vi "Graphe_XY.vi"(0 "Graphe":T1(graph), 3 "Tableau de chaînes":string[](array[string])) -> ()   [LabVIEW 2015]
uses:
  <vilib>/Utility/miscctls.llb/LVPositionTypeDef.ctl
panel:
  out "Calculs maths":dbl[](array[numeric])
  in  "Bouton Aide":bool
  in  "=":string
  in  "Selec Maths":u16(ring) caption="Maintenir la touche CTRL appuyée pour tout afficher" items=["Moyenne", "Min", "Max", "Ecart type", "Variance", "Intégrale", "Pente ajust. lin.", "Offset ajust. lin.", "Résidus ajust. lin.", "R²", "Amplitude ajust. exp", "Atténuation ajust. exp", "Offset ajust. exp", "Résidus ajust. exp"]
  in  "Active maths":bool
  out "Valeur maths":dbl
  out "Nbre courbes":i32
  in  "Quitter graphe":bool
  in  "Palette:Outil actif":i32
  in  "Curseur visible":bool
  in  "Tout sélectionner":bool
  in  "Curseur":u16(ring) items=["2", "3", "4", "5", "6", "7", "8"]
  in  "Quadrillage":u16(ring)=1 items=["Sans", "Horizontal", "Vertical", "Tout"]
  in  "Mini":dbl max=19.999 format="%#.3f"
  in  "Maxi":dbl min=0.001 format="%#.3f"
  in  "Echelle Y":u16(ring) items=["Manu"=0, "Auto"=2]
  out "Y":dbl
  out "X":timestamp format="%<%.3X>T"
  # "="
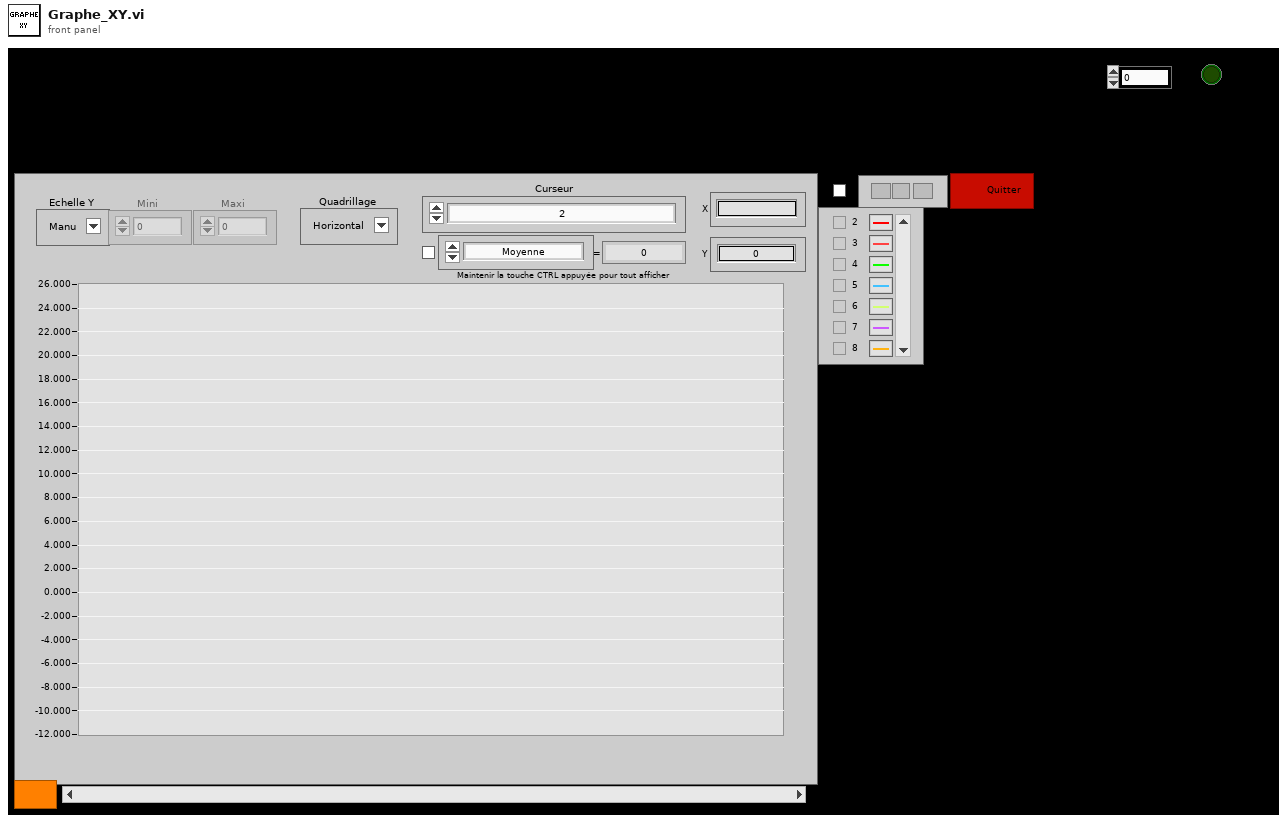
[diagram p1: front panel]
types:
  T1 = cluster{"Horodatage":timestamp[], "Donnees":dbl[]}[]
  T2 = typedef "LVPositionTypeDef.ctl" = cluster{"Left":i32, "Top":i32}
  T3 = cluster{"Shift":bool, "Ctrl":bool, "Alt":bool, "Cmd":bool, "Opt":bool}
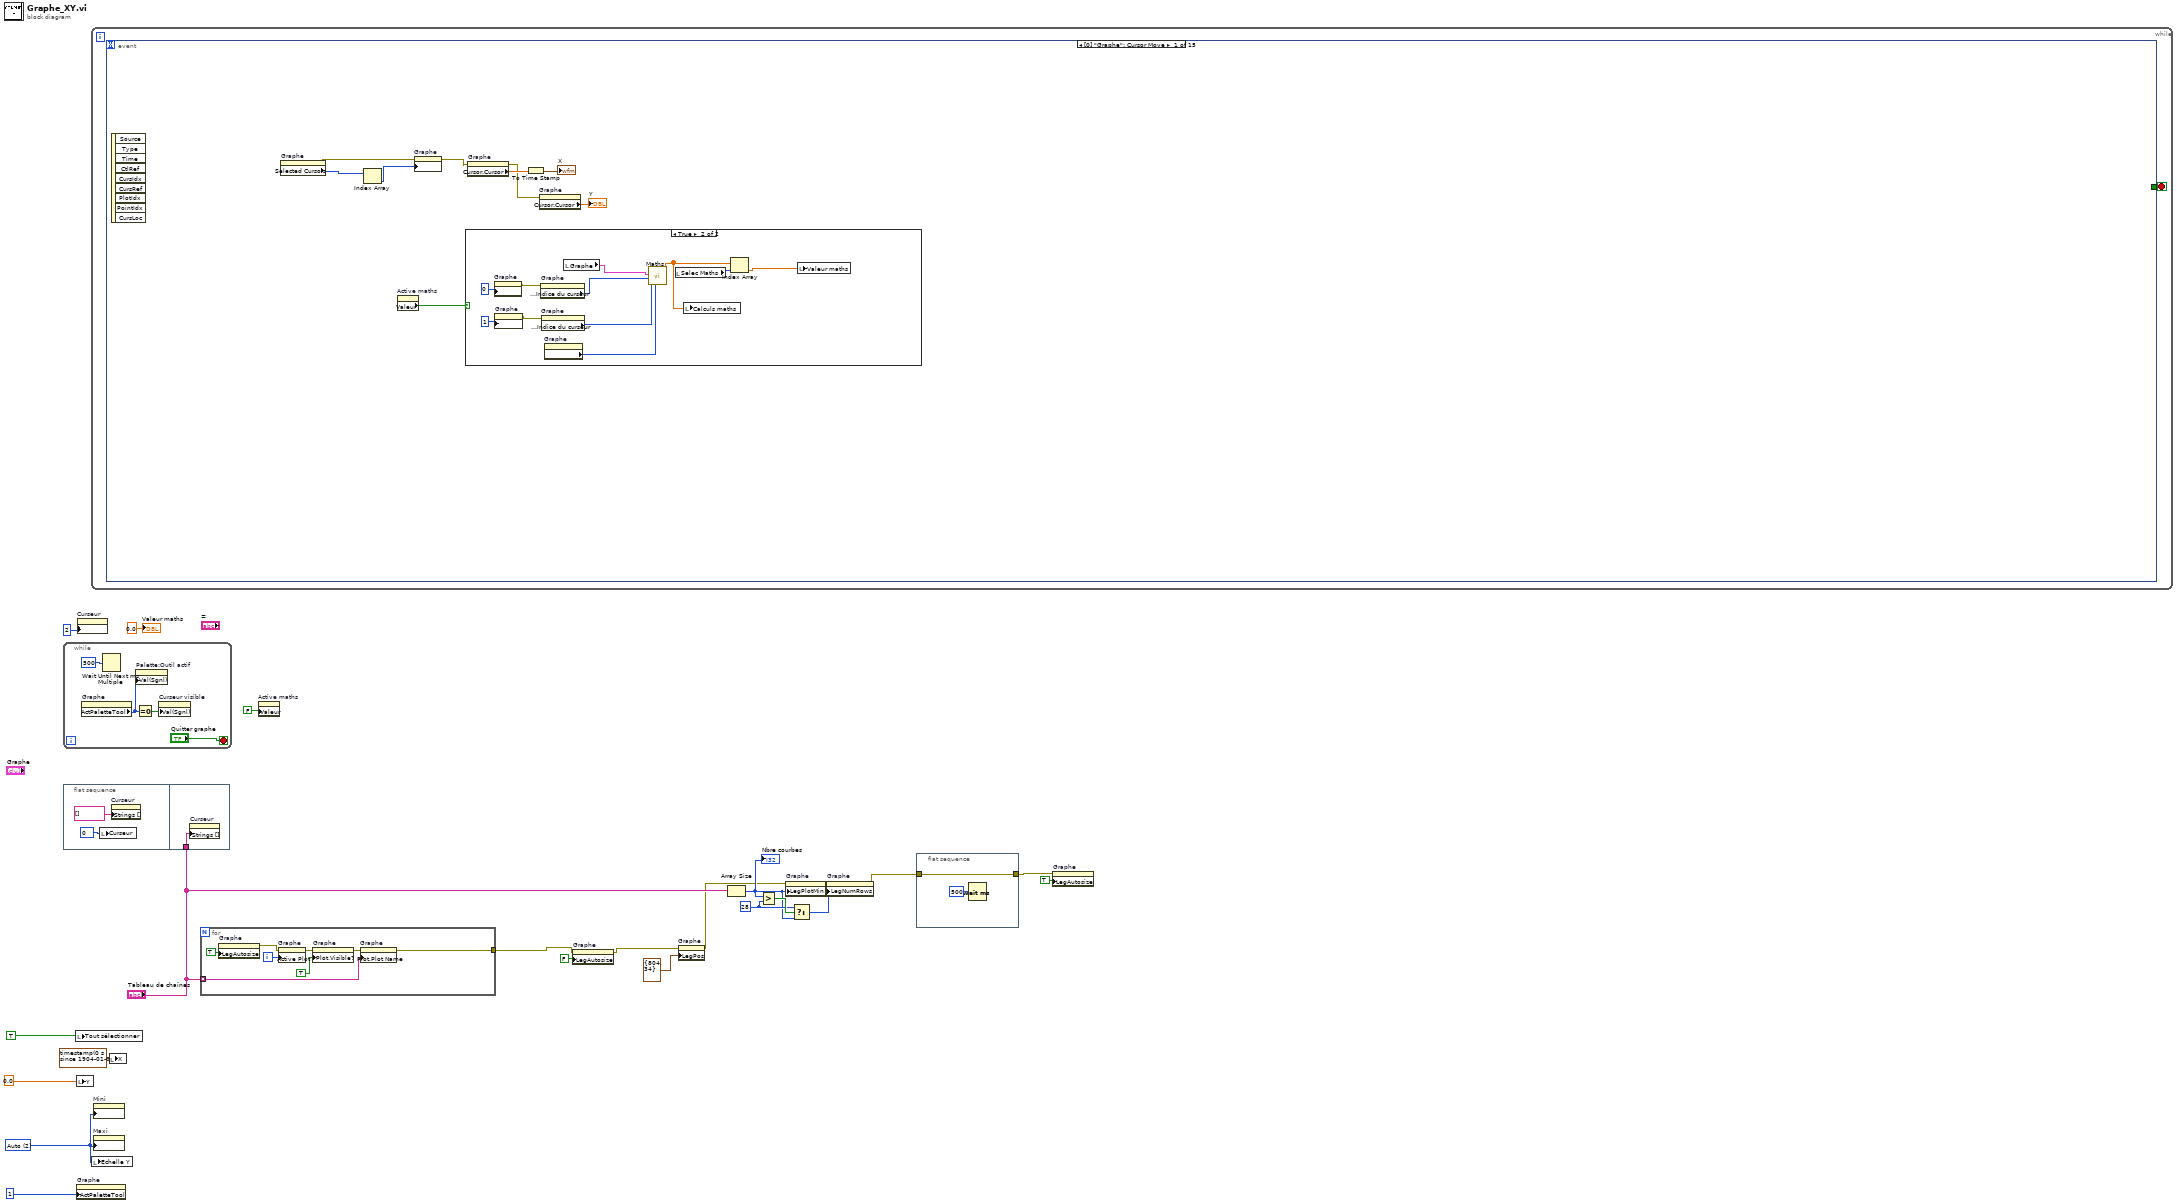
[diagram p0: block diagram]
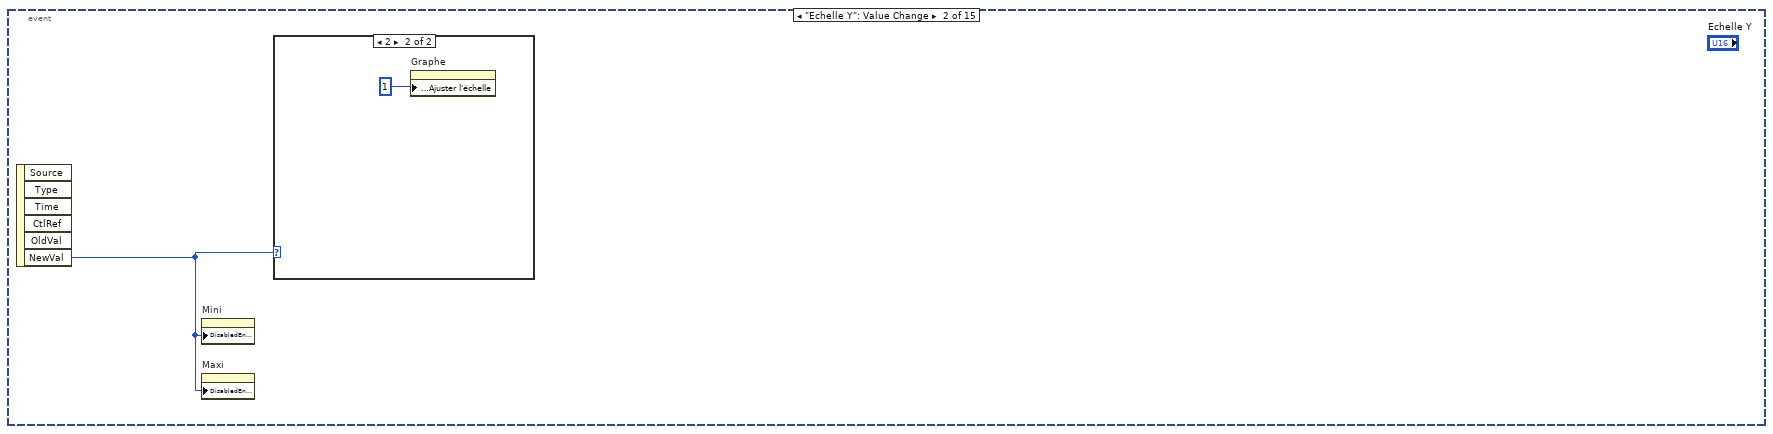
[diagram p3: hidden frame]
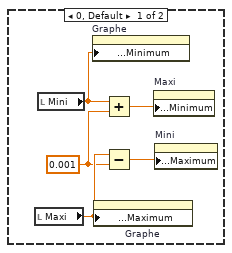
[diagram p4: hidden frame]
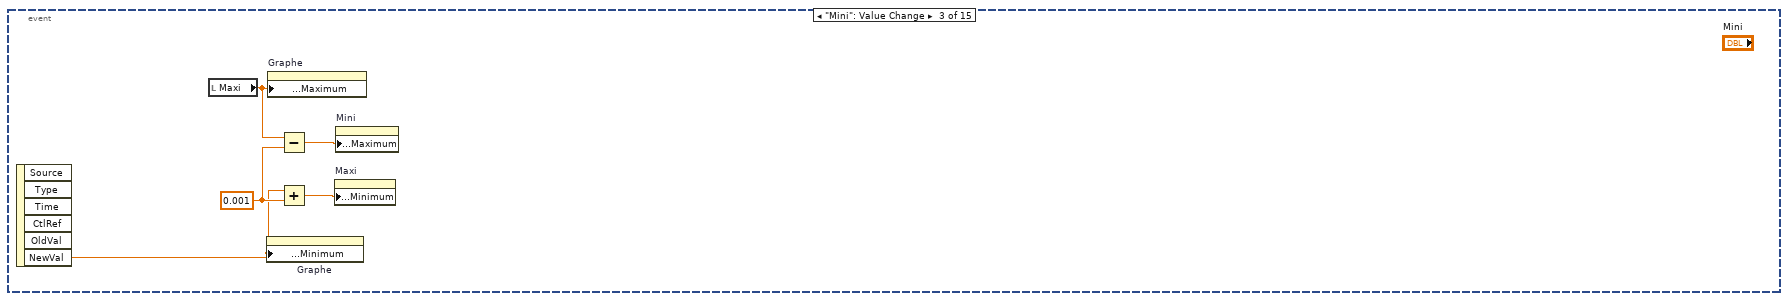
[diagram p5: hidden frame]
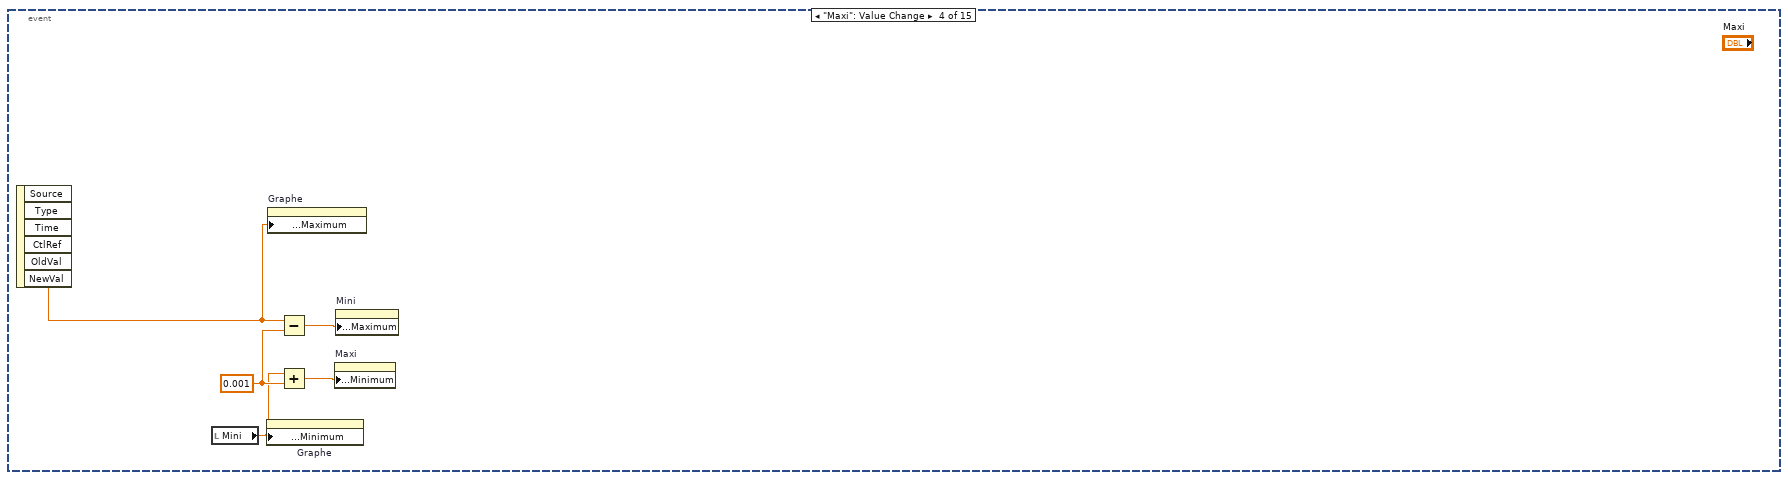
[diagram p6: hidden frame]
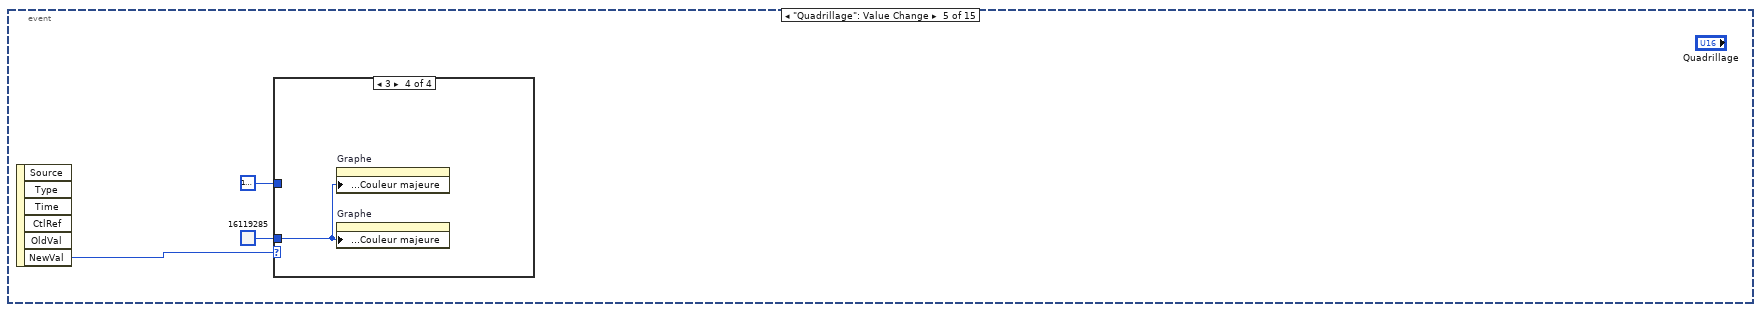
[diagram p7: hidden frame]
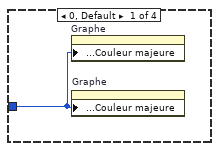
[diagram p8: hidden frame]
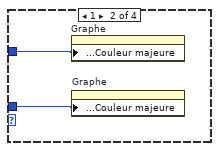
[diagram p9: hidden frame]
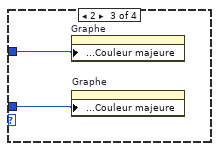
[diagram p10: hidden frame]
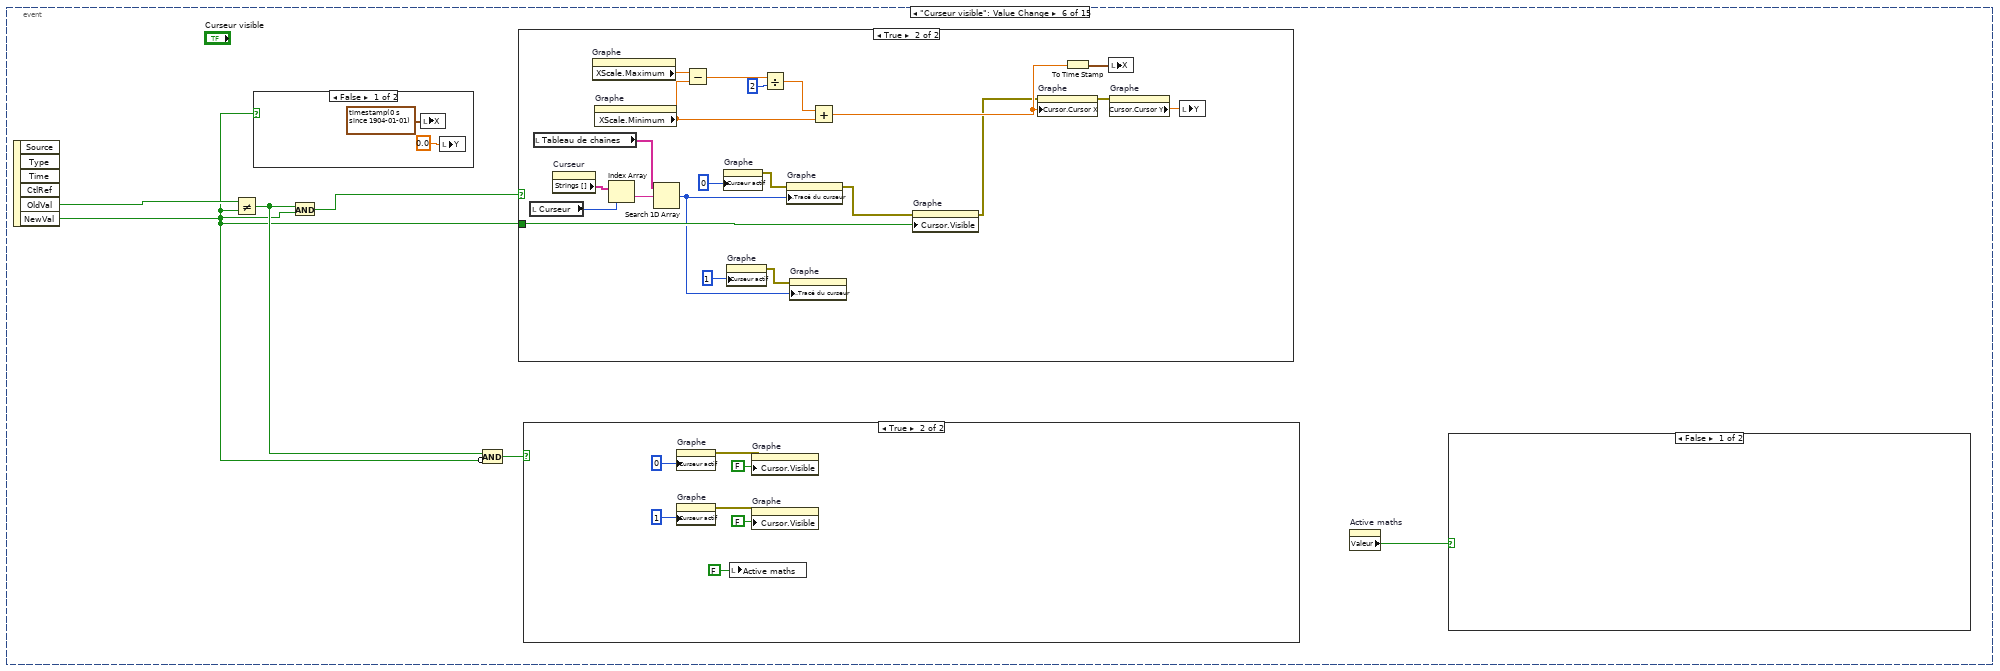
[diagram p11: hidden frame]
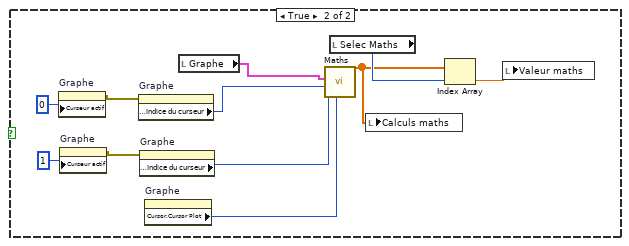
[diagram p12: hidden frame]
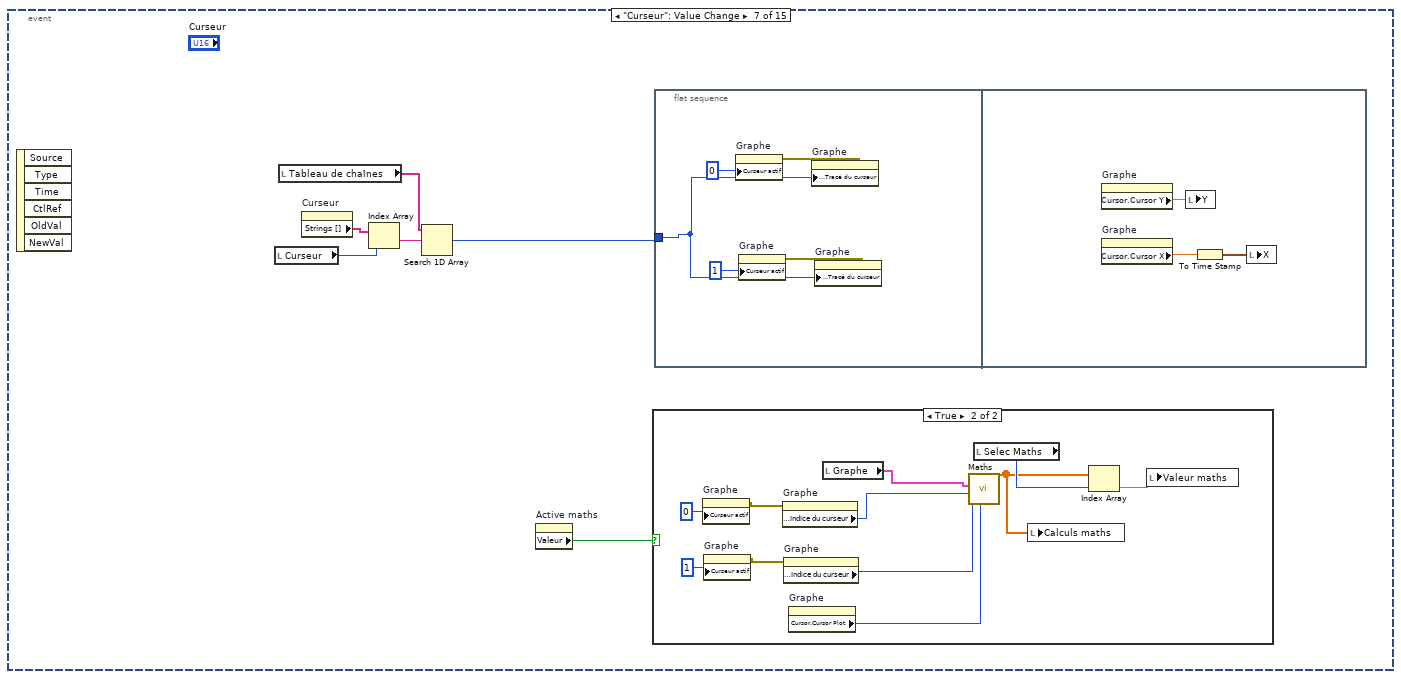
[diagram p16: hidden frame]
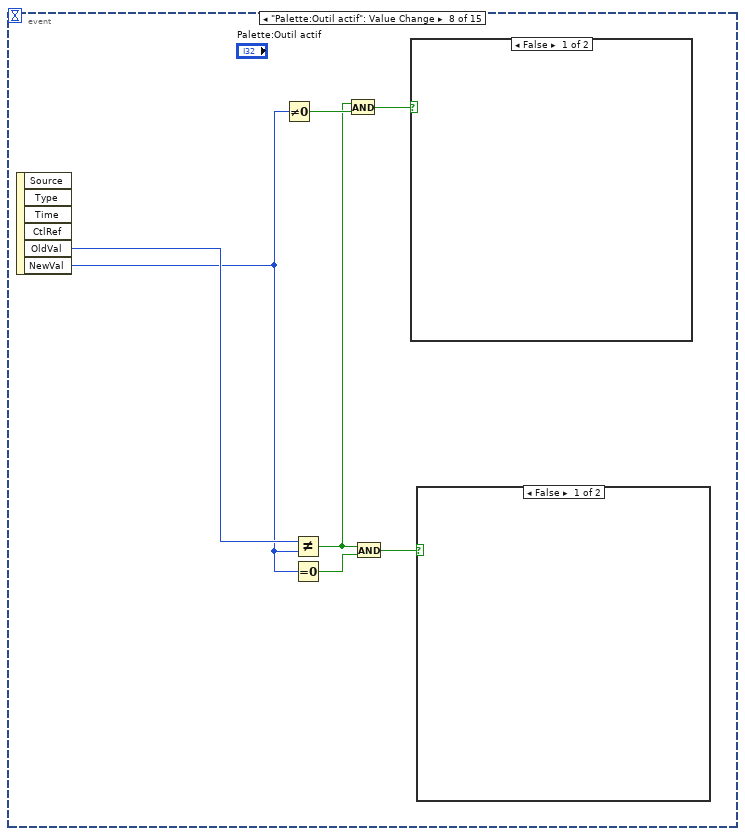
[diagram p18: hidden frame]
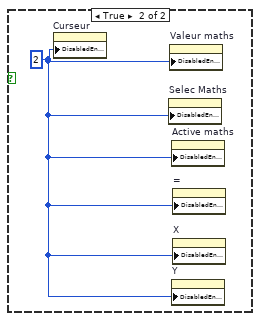
[diagram p19: hidden frame]
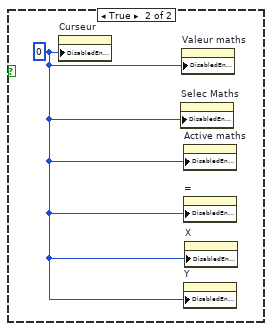
[diagram p20: hidden frame]
diagram:
  w13 = 28 ("y")
  w22 = u16 2 items=["Manu"=0, "Auto"=2] ("Echelle Y")
  n1 = while {
    stop <- "Quitter graphe" stop-if-true
    n2 = property on="Graphe" class="XYGraph (strict)"() -> ("ActPaletteTool"=w24:i32)  [unwired: 2 in, 2 out]
    n3 = Wait Until Next ms Multiple(millisecond multiple=u32 500 ("n millisecondes")) -> ()  [unwired: 1 out]
    n4 = property on="Palette:Outil actif" class="DigNum (strict)"("Val(Sgnl)"=w24) -> ()  [unwired: 2 in, 2 out]
    n5 = Equal To 0?(x=w24) -> (x = 0?=w25:bool)
    n6 = property on="Curseur visible" class="Bool (strict)"("Val(Sgnl)"=w25) -> ()  [unwired: 2 in, 2 out]
  }
  n7 = flat-sequence {
    tunnel: "Tableau de chaînes" -> [w29]
    frame #0 {
      w28 = u16 0 items=[""] ("Curseur")
      n8 = local write "Curseur"(w28) -> ()
      n9 = property on="Curseur" class="Ring (strict)"("Strings []"=string[] [] ("Chaînes []")) -> ()  [unwired: 2 in, 2 out]
    }
    frame #1 {
      n10 = property on="Curseur" class="Ring (strict)"("Strings []"=w29) -> ()  [unwired: 2 in, 2 out]
    }
  }
  n11 = local write "Tout sélectionner"(TRUE ("Tout sélectionner")) -> ()
  n12 = local write "Y"(0.0 ("Y")) -> ()
  n13 = property on="Graphe" class="XYGraph (strict)"("ActPaletteTool"=1 ("Palette:Outil actif")) -> ()  [unwired: 2 in, 2 out]
  n14 = property on="Curseur" class="Ring (strict)"("DisabledEnum"=i8 2 ("cas vrai")) -> ()  [unwired: 2 in, 2 out]
  n15 = while {
    stop <- w30 stop-if-true
    n16 = event shown="[0] \"Graphe\": Cursor Move" {
      selector: _ -> [_ _ _ _ _ _ _ _ _ _ _ _ _ _ _]
      dyn-events: _ -> [_ _ _ _ _ _ _ _ _ _ _ _ _ _ _]
      timeout: _ -> [_ _ _ _ _ _ _ _ _ _ _ _ _ _ _]
      tunnel: [_ _ _ _ _ _ _ _ _ _ _ _ _ w275 _] -> w30
      event "Graphe": Cursor Move {
        n17 = event-data() -> ()  [unwired: 1 in, 9 out]
        n18 = property on="Graphe" class="XYGraph (strict)"() -> (error out=w33:errorcluster, "Selected Cursors"=w35:u32[])  [unwired: 2 in, 1 out]
        n19 = Index Array(array=w35) -> (element=w34:u32)  [unwired: 1 in]
        n20 = property on="Active maths" class="Bool (strict)"() -> ("Valeur"=w31:bool)  [unwired: 2 in, 2 out]
        n21 = property on="Graphe" class="XYGraph (strict)"(error in=w33, "Active Cursor"=w34) -> (error out=w32:errorcluster)  [unwired: 1 in, 1 out]
        n22 = case shown="True" w31 {
          frame False {
          }
          frame True {
            n23 = property on="Graphe" class="XYGraph (strict)"("Curseur actif"=u32 0) -> (error out=w50:errorcluster)  [unwired: 2 in, 1 out]
            n24 = property on="Graphe" class="XYGraph (strict)"("Curseur actif"=u32 1) -> (error out=w46:errorcluster)  [unwired: 2 in, 1 out]
            n25 = property on="Graphe" class="XYGraph (strict)"(error in=w50) -> ("Curseur.Indice du curseur"=w48:i32)  [unwired: 1 in, 2 out]
            n26 = property on="Graphe" class="XYGraph (strict)"(error in=w46) -> ("Curseur.Indice du curseur"=w45:i32)  [unwired: 1 in, 2 out]
            n27 = property on="Graphe" class="XYGraph (strict)"() -> ("Cursor.Cursor Plot"=w44:i32)  [unwired: 2 in, 2 out]
            n28 = local read "Graphe"() -> (w43:T1)
            n29 = call "Maths.vi"("Curseur tracé"=w44, "Indice curseur 2"=w45, "Indice curseur 1"=w48, "Graphe"=w43) -> ("Calculs maths"=w40:dbl[])  [unwired: 7 in]
            n30 = local read "Selec Maths"() -> (w41:u16)
            n31 = local write "Calculs maths"(w40) -> ()
            n32 = Index Array(array=w40, index=w41) -> (element=w42:dbl)
            n33 = local write "Valeur maths"(w42) -> ()
          }
        }
        n34 = property on="Graphe" class="XYGraph (strict)"(error in=w32) -> (error out=w36:errorcluster, "Cursor.Cursor X"=w38:dbl)  [unwired: 1 in, 1 out]
        n35 = To Time Stamp(1:w38) -> (0:→"X":timestamp)
        n36 = property on="Graphe" class="XYGraph (strict)"(error in=w36) -> ("Cursor.Cursor Y"=→"Y":dbl)  [unwired: 1 in, 2 out]
      }
      event "Echelle Y": Value Change {
        n37 = event-data() -> ("NewVal"=w51:u16)  [unwired: 1 in, 5 out]
        n38 = property on="Mini" class="DigNum (strict)"("DisabledEnum"=w51) -> ()  [unwired: 2 in, 2 out]
        n39 = property on="Maxi" class="DigNum (strict)"("DisabledEnum"=w51) -> ()  [unwired: 2 in, 2 out]
        n40 = case shown="2" w51 {
          frame 0, Default {
            w55 = 0.001 ("y")
            n41 = local read "Maxi"() -> (w56:dbl)
            n42 = local read "Mini"() -> (w52:dbl)
            n43 = property on="Graphe" class="XYGraph (strict)"("Échelle des Y.Gamme:Minimum"=w52) -> ()  [unwired: 2 in, 2 out]
            n44 = property on="Graphe" class="XYGraph (strict)"("Échelle des Y.Gamme:Maximum"=w56) -> ()  [unwired: 2 in, 2 out]
            n45 = Add(x=w52, y=w55) -> (x+y=w53:dbl)
            n46 = Subtract(x=w56, y=w55) -> (x-y=w54:dbl)
            n47 = property on="Maxi" class="DigNum (strict)"("Limites d'entrée des données:Minimum"=w53) -> ()  [unwired: 2 in, 2 out]
            n48 = property on="Mini" class="DigNum (strict)"("Limites d'entrée des données:Maximum"=w54) -> ()  [unwired: 2 in, 2 out]
          }
          frame 2 {
            n49 = property on="Graphe" class="XYGraph (strict)"("Échelle des Y.Ajuster l'échelle"=u8 1 ("Échelle Y.Ajuster l'échelle")) -> ()  [unwired: 2 in, 2 out]
          }
        }
      }
      event "Mini": Value Change {
        w61 = 0.001 ("y")
        n50 = event-data() -> ("NewVal"=w58:dbl)  [unwired: 1 in, 5 out]
        n51 = local read "Maxi"() -> (w62:dbl)
        n52 = property on="Graphe" class="XYGraph (strict)"("Échelle des Y.Gamme:Minimum"=w58) -> ()  [unwired: 2 in, 2 out]
        n53 = property on="Graphe" class="XYGraph (strict)"("Échelle des Y.Gamme:Maximum"=w62) -> ()  [unwired: 2 in, 2 out]
        n54 = Subtract(x=w62, y=w61) -> (x-y=w60:dbl)
        n55 = Add(x=w58, y=w61) -> (x+y=w59:dbl)
        n56 = property on="Maxi" class="DigNum (strict)"("Limites d'entrée des données:Minimum"=w59) -> ()  [unwired: 2 in, 2 out]
        n57 = property on="Mini" class="DigNum (strict)"("Limites d'entrée des données:Maximum"=w60) -> ()  [unwired: 2 in, 2 out]
      }
      event "Maxi": Value Change {
        w67 = 0.001 ("y")
        n58 = event-data() -> ("NewVal"=w64:dbl)  [unwired: 1 in, 5 out]
        n59 = local read "Mini"() -> (w63:dbl)
        n60 = property on="Graphe" class="XYGraph (strict)"("Échelle des Y.Gamme:Minimum"=w63) -> ()  [unwired: 2 in, 2 out]
        n61 = property on="Graphe" class="XYGraph (strict)"("Échelle des Y.Gamme:Maximum"=w64) -> ()  [unwired: 2 in, 2 out]
        n62 = Subtract(x=w64, y=w67) -> (x-y=w66:dbl)
        n63 = Add(x=w63, y=w67) -> (x+y=w65:dbl)
        n64 = property on="Maxi" class="DigNum (strict)"("Limites d'entrée des données:Minimum"=w65) -> ()  [unwired: 2 in, 2 out]
        n65 = property on="Mini" class="DigNum (strict)"("Limites d'entrée des données:Maximum"=w66) -> ()  [unwired: 2 in, 2 out]
      }
      event "Quadrillage": Value Change {
        n66 = event-data() -> ("NewVal"=w70:u16)  [unwired: 1 in, 5 out]
        n67 = case shown="3" w70 {
          tunnel: u32 16119285 -> [_ w73 w75 w76]
          tunnel: u32 16777216 -> [w71 w72 w74 _]
          frame 0, Default {
            n68 = property on="Graphe" class="XYGraph (strict)"("Échelle des X.Couleurs de grille:Couleur majeure"=w71) -> ()  [unwired: 2 in, 2 out]
            n69 = property on="Graphe" class="XYGraph (strict)"("Échelle des Y.Couleurs de grille:Couleur majeure"=w71) -> ()  [unwired: 2 in, 2 out]
          }
          frame 1 {
            n70 = property on="Graphe" class="XYGraph (strict)"("Échelle des X.Couleurs de grille:Couleur majeure"=w72) -> ()  [unwired: 2 in, 2 out]
            n71 = property on="Graphe" class="XYGraph (strict)"("Échelle des Y.Couleurs de grille:Couleur majeure"=w73) -> ()  [unwired: 2 in, 2 out]
          }
          frame 2 {
            n72 = property on="Graphe" class="XYGraph (strict)"("Échelle des Y.Couleurs de grille:Couleur majeure"=w74) -> ()  [unwired: 2 in, 2 out]
            n73 = property on="Graphe" class="XYGraph (strict)"("Échelle des X.Couleurs de grille:Couleur majeure"=w75) -> ()  [unwired: 2 in, 2 out]
          }
          frame 3 {
            n74 = property on="Graphe" class="XYGraph (strict)"("Échelle des X.Couleurs de grille:Couleur majeure"=w76) -> ()  [unwired: 2 in, 2 out]
            n75 = property on="Graphe" class="XYGraph (strict)"("Échelle des Y.Couleurs de grille:Couleur majeure"=w76) -> ()  [unwired: 2 in, 2 out]
          }
        }
      }
      event "Curseur visible": Value Change {
        n76 = event-data() -> ("OldVal"=w82:bool, "NewVal"=w78:bool)  [unwired: 1 in, 4 out]
        n77 = Not Equal?(x=w82, y=w78) -> (x != y?=w80:bool)
        n78 = case shown="False" w78 {
          frame False {
            n79 = local write "X"(timestamp(0 s since 1904-01-01) ("X")) -> ()
            n80 = local write "Y"(0.0 ("Y")) -> ()
          }
          frame True {
          }
        }
        n81 = And(x=w80, y=w78) -> (x .and. y?=w81:bool)
        n82 = Compound Arithmetic op=AND(w80, invert w78) -> (w79:bool)
        n83 = case shown="True" w81 {
          tunnel: w78 -> [_ w113]
          frame False {
          }
          frame True {
            n84 = local read "Curseur"() -> (w108:u16)
            n85 = local read "Tableau de chaînes"() -> (w111:string[])
            n86 = property on="Curseur" class="Ring (strict)"() -> ("Strings []"=w109:string[])  [unwired: 2 in, 2 out]
            n87 = property on="Graphe" class="XYGraph (strict)"() -> ("XScale.Maximum"=w122:dbl)  [unwired: 2 in, 2 out]
            n88 = property on="Graphe" class="XYGraph (strict)"() -> ("XScale.Minimum"=w119:dbl)  [unwired: 2 in, 2 out]
            n89 = Index Array(array=w109, index=w108) -> (element=w110:string)
            n90 = Search 1D Array(1D array=w111, element=w110) -> (index of element=w105:i32)  [unwired: 1 in]
            n91 = Subtract(x=w122, y=w119) -> (x-y=w121:dbl)
            n92 = property on="Graphe" class="XYGraph (strict)"("Curseur actif"=u32 0) -> (error out=w112:errorcluster)  [unwired: 2 in, 1 out]
            n93 = property on="Graphe" class="XYGraph (strict)"("Curseur actif"=u32 1) -> (error out=w107:errorcluster)  [unwired: 2 in, 1 out]
            n94 = Divide(x=w121, y=2) -> (x/y=w120:dbl)
            n95 = property on="Graphe" class="XYGraph (strict)"(error in=w112, "Curseur.Tracé du curseur"=w105) -> (error out=w103:errorcluster)  [unwired: 1 in, 1 out]
            n96 = property on="Graphe" class="XYGraph (strict)"(error in=w107, "Curseur.Tracé du curseur"=w105) -> ()  [unwired: 1 in, 2 out]
            n97 = Add(x=w120, y=w119) -> (x+y=w116:dbl)
            n98 = property on="Graphe" class="XYGraph (strict)"(error in=w103, "Cursor.Visible"=w113) -> (error out=w104:errorcluster)  [unwired: 1 in, 1 out]
            n99 = property on="Graphe" class="XYGraph (strict)"(error in=w104, "Cursor.Cursor X"=w116) -> (error out=w115:errorcluster)  [unwired: 1 in, 1 out]
            n100 = To Time Stamp(1:w116) -> (0:w117:timestamp)
            n101 = local write "X"(w117) -> ()
            n102 = property on="Graphe" class="XYGraph (strict)"(error in=w115) -> ("Cursor.Cursor Y"=w118:dbl)  [unwired: 1 in, 2 out]
            n103 = local write "Y"(w118) -> ()
          }
        }
        n104 = case shown="True" w79 {
          frame False {
          }
          frame True {
            n105 = property on="Graphe" class="XYGraph (strict)"("Curseur actif"=u32 0) -> (error out=w99:errorcluster)  [unwired: 2 in, 1 out]
            n106 = property on="Graphe" class="XYGraph (strict)"("Curseur actif"=u32 1) -> (error out=w96:errorcluster)  [unwired: 2 in, 1 out]
            n107 = local write "Active maths"(FALSE ("Selection math")) -> ()
            n108 = property on="Graphe" class="XYGraph (strict)"(error in=w99, "Cursor.Visible"=FALSE ("Curseur.Visible")) -> ()  [unwired: 1 in, 2 out]
            n109 = property on="Graphe" class="XYGraph (strict)"(error in=w96, "Cursor.Visible"=FALSE ("Curseur.Visible")) -> ()  [unwired: 1 in, 2 out]
          }
        }
        n110 = property on="Active maths" class="Bool (strict)"() -> ("Valeur"=w77:bool)  [unwired: 2 in, 2 out]
        n111 = case shown="False" w77 {
          frame False {
          }
          frame True {
            n112 = property on="Graphe" class="XYGraph (strict)"("Curseur actif"=u32 0) -> (error out=w93:errorcluster)  [unwired: 2 in, 1 out]
            n113 = property on="Graphe" class="XYGraph (strict)"("Curseur actif"=u32 1) -> (error out=w89:errorcluster)  [unwired: 2 in, 1 out]
            n114 = property on="Graphe" class="XYGraph (strict)"(error in=w93) -> ("Curseur.Indice du curseur"=w91:i32)  [unwired: 1 in, 2 out]
            n115 = property on="Graphe" class="XYGraph (strict)"(error in=w89) -> ("Curseur.Indice du curseur"=w88:i32)  [unwired: 1 in, 2 out]
            n116 = property on="Graphe" class="XYGraph (strict)"() -> ("Cursor.Cursor Plot"=w87:i32)  [unwired: 2 in, 2 out]
            n117 = local read "Graphe"() -> (w86:T1)
            n118 = call "Maths.vi"("Curseur tracé"=w87, "Indice curseur 2"=w88, "Indice curseur 1"=w91, "Graphe"=w86) -> ("Calculs maths"=w83:dbl[])  [unwired: 7 in]
            n119 = local read "Selec Maths"() -> (w85:u16)
            n120 = local write "Calculs maths"(w83) -> ()
            n121 = Index Array(array=w83, index=w85) -> (element=w84:dbl)
            n122 = local write "Valeur maths"(w84) -> ()
          }
        }
      }
      event "Curseur": Value Change {
        n123 = event-data() -> ()  [unwired: 1 in, 6 out]
        n124 = local read "Curseur"() -> (w125:u16)
        n125 = local read "Tableau de chaînes"() -> (w128:string[])
        n126 = property on="Curseur" class="Ring (strict)"() -> ("Strings []"=w126:string[])  [unwired: 2 in, 2 out]
        n127 = Index Array(array=w126, index=w125) -> (element=w127:string)
        n128 = Search 1D Array(1D array=w128, element=w127) -> (index of element=w124:i32)  [unwired: 1 in]
        n129 = property on="Active maths" class="Bool (strict)"() -> ("Valeur"=w129:bool)  [unwired: 2 in, 2 out]
        n130 = case shown="True" w129 {
          frame False {
          }
          frame True {
            n131 = property on="Graphe" class="XYGraph (strict)"("Curseur actif"=u32 0) -> (error out=w140:errorcluster)  [unwired: 2 in, 1 out]
            n132 = property on="Graphe" class="XYGraph (strict)"("Curseur actif"=u32 1) -> (error out=w136:errorcluster)  [unwired: 2 in, 1 out]
            n133 = property on="Graphe" class="XYGraph (strict)"(error in=w140) -> ("Curseur.Indice du curseur"=w138:i32)  [unwired: 1 in, 2 out]
            n134 = property on="Graphe" class="XYGraph (strict)"(error in=w136) -> ("Curseur.Indice du curseur"=w135:i32)  [unwired: 1 in, 2 out]
            n135 = property on="Graphe" class="XYGraph (strict)"() -> ("Cursor.Cursor Plot"=w134:i32)  [unwired: 2 in, 2 out]
            n136 = local read "Graphe"() -> (w133:T1)
            n137 = call "Maths.vi"("Curseur tracé"=w134, "Indice curseur 2"=w135, "Indice curseur 1"=w138, "Graphe"=w133) -> ("Calculs maths"=w130:dbl[])  [unwired: 7 in]
            n138 = local read "Selec Maths"() -> (w132:u16)
            n139 = local write "Calculs maths"(w130) -> ()
            n140 = Index Array(array=w130, index=w132) -> (element=w131:dbl)
            n141 = local write "Valeur maths"(w131) -> ()
          }
        }
        n142 = flat-sequence {
          tunnel: w124 -> [w141]
          frame #0 {
            n143 = property on="Graphe" class="XYGraph (strict)"("Curseur actif"=u32 0) -> (error out=w144:errorcluster)  [unwired: 2 in, 1 out]
            n144 = property on="Graphe" class="XYGraph (strict)"("Curseur actif"=u32 1) -> (error out=w143:errorcluster)  [unwired: 2 in, 1 out]
            n145 = property on="Graphe" class="XYGraph (strict)"(error in=w144, "Curseur.Tracé du curseur"=w141) -> ()  [unwired: 1 in, 2 out]
            n146 = property on="Graphe" class="XYGraph (strict)"(error in=w143, "Curseur.Tracé du curseur"=w141) -> ()  [unwired: 1 in, 2 out]
          }
          frame #1 {
            n147 = property on="Graphe" class="XYGraph (strict)"() -> ("Cursor.Cursor Y"=w148:dbl)  [unwired: 2 in, 2 out]
            n148 = property on="Graphe" class="XYGraph (strict)"() -> ("Cursor.Cursor X"=w146:dbl)  [unwired: 2 in, 2 out]
            n149 = local write "Y"(w148) -> ()
            n150 = To Time Stamp(1:w146) -> (0:w147:timestamp)
            n151 = local write "X"(w147) -> ()
          }
        }
      }
      event "Palette:Outil actif": Value Change {
        n152 = event-data() -> ("OldVal"=w155:i32, "NewVal"=w151:i32)  [unwired: 1 in, 4 out]
        n153 = Not Equal To 0?(x=w151) -> (x != 0?=w152:bool)
        n154 = Not Equal?(x=w155, y=w151) -> (x != y?=w150:bool)
        n155 = Equal To 0?(x=w151) -> (x = 0?=w149:bool)
        n156 = And(x=w150, y=w152) -> (x .and. y?=w153:bool)
        n157 = And(x=w150, y=w149) -> (x .and. y?=w154:bool)
        n158 = case shown="False" w153 {
          frame False {
          }
          frame True {
            w156 = i8 2 ("cas vrai")
            n159 = property on="Curseur" class="Ring (strict)"("DisabledEnum"=w156) -> ()  [unwired: 2 in, 2 out]
            n160 = property on="Selec Maths" class="Ring (strict)"("DisabledEnum"=w156) -> ()  [unwired: 2 in, 2 out]
            n161 = property on="Valeur maths" class="DigNum (strict)"("DisabledEnum"=w156) -> ()  [unwired: 2 in, 2 out]
            n162 = property on="Active maths" class="Bool (strict)"("DisabledEnum"=w156) -> ()  [unwired: 2 in, 2 out]
            n163 = property on="Y" class="DigNum (strict)"("DisabledEnum"=w156) -> ()  [unwired: 2 in, 2 out]
            n164 = property on="=" class="Str"("DisabledEnum"=w156) -> ()  [unwired: 2 in, 2 out]
            n165 = property on="X" class="AbsTime (strict)"("DisabledEnum"=w156) -> ()  [unwired: 2 in, 2 out]
          }
        }
        n166 = case shown="False" w154 {
          frame False {
          }
          frame True {
            w157 = i8 0 ("cas vrai")
            n167 = property on="Curseur" class="Ring (strict)"("DisabledEnum"=w157) -> ()  [unwired: 2 in, 2 out]
            n168 = property on="Selec Maths" class="Ring (strict)"("DisabledEnum"=w157) -> ()  [unwired: 2 in, 2 out]
            n169 = property on="Valeur maths" class="DigNum (strict)"("DisabledEnum"=w157) -> ()  [unwired: 2 in, 2 out]
            n170 = property on="Active maths" class="Bool (strict)"("DisabledEnum"=w157) -> ()  [unwired: 2 in, 2 out]
            n171 = property on="=" class="Str"("DisabledEnum"=w157) -> ()  [unwired: 2 in, 2 out]
            n172 = property on="Y" class="DigNum (strict)"("DisabledEnum"=w157) -> ()  [unwired: 2 in, 2 out]
            n173 = property on="X" class="AbsTime (strict)"("DisabledEnum"=w157) -> ()  [unwired: 2 in, 2 out]
          }
        }
      }
      event "Active maths": Value Change {
        n174 = event-data() -> ("OldVal"=w166:bool, "NewVal"=w165:bool)  [unwired: 1 in, 4 out]
        n175 = property on="Curseur visible" class="Bool (strict)"() -> ("Value"=w163:bool)  [unwired: 2 in, 2 out]
        n176 = property on="Active maths" class="Bool (strict)"() -> ("Valeur"=w158:bool)  [unwired: 2 in, 2 out]
        n177 = case shown="False" w165 {
          frame False {
            n178 = local write "Valeur maths"(0.0 ("Valeur Moyenne")) -> ()
          }
          frame True {
          }
        }
        n179 = case shown="True" w158 {
          frame False {
          }
          frame True {
            n180 = property on="Graphe" class="XYGraph (strict)"("Curseur actif"=u32 0) -> (error out=w179:errorcluster)  [unwired: 2 in, 1 out]
            n181 = property on="Graphe" class="XYGraph (strict)"("Curseur actif"=u32 1) -> (error out=w175:errorcluster)  [unwired: 2 in, 1 out]
            n182 = property on="Graphe" class="XYGraph (strict)"(error in=w179) -> ("Curseur.Indice du curseur"=w177:i32)  [unwired: 1 in, 2 out]
            n183 = property on="Graphe" class="XYGraph (strict)"(error in=w175) -> ("Curseur.Indice du curseur"=w174:i32)  [unwired: 1 in, 2 out]
            n184 = property on="Graphe" class="XYGraph (strict)"() -> ("Cursor.Cursor Plot"=w173:i32)  [unwired: 2 in, 2 out]
            n185 = local read "Graphe"() -> (w172:T1)
            n186 = call "Maths.vi"("Curseur tracé"=w173, "Indice curseur 2"=w174, "Indice curseur 1"=w177, "Graphe"=w172) -> ("Calculs maths"=w169:dbl[])  [unwired: 7 in]
            n187 = local read "Selec Maths"() -> (w170:u16)
            n188 = local write "Calculs maths"(w169) -> ()
            n189 = Index Array(array=w169, index=w170) -> (element=w171:dbl)
            n190 = local write "Valeur maths"(w171) -> ()
          }
        }
        n191 = Not Equal?(x=w166, y=w165) -> (x != y?=w168:bool)
        n192 = And(x=w163, y=w158) -> (x .and. y?=w167:bool)
        n193 = property on="Graphe" class="XYGraph (strict)"("Curseur actif"=u32 0) -> (error out=w160:errorcluster)  [unwired: 2 in, 1 out]
        n194 = property on="Graphe" class="XYGraph (strict)"(error in=w160, "Curseur.Visible"=w163) -> (error out=w162:errorcluster)  [unwired: 1 in, 1 out]
        n195 = property on="Graphe" class="XYGraph (strict)"(error in=w162, "Curseur actif"=u32 1) -> (error out=w159:errorcluster)  [unwired: 1 in, 1 out]
        n196 = property on="Graphe" class="XYGraph (strict)"(error in=w159, "Curseur.Visible"=w167) -> ()  [unwired: 1 in, 2 out]
        n197 = flat-sequence {
          tunnel: w168 -> [w180]
          frame #0 {
            n198 = case shown="True" w180 {
              frame False {
              }
              frame True {
                n199 = property on="Graphe" class="XYGraph (strict)"() -> ("Échelle des X.Gamme:Maximum"=w183:dbl)  [unwired: 2 in, 2 out]
                n200 = property on="Graphe" class="XYGraph (strict)"() -> ("Échelle des X.Gamme:Minimum"=w185:dbl)  [unwired: 2 in, 2 out]
                n201 = Subtract(x=w183, y=w185) -> (x-y=w182:dbl)
                n202 = Divide(x=w182, y=2.0) -> (x/y=w184:dbl)
                n203 = Add(x=w184, y=w185) -> (x+y=w186:dbl)
                n204 = property on="Graphe" class="XYGraph (strict)"("Curseur.Position du curseur:Curseur X"=w186) -> ()  [unwired: 2 in, 2 out]
              }
            }
          }
        }
      }
      event "Selec Maths": Value Change {
        n205 = event-data() -> ()  [unwired: 1 in, 6 out]
        n206 = property on="Active maths" class="Bool (strict)"() -> ("Valeur"=w188:bool)  [unwired: 2 in, 2 out]
        n207 = case shown="True" w188 {
          frame False {
          }
          frame True {
            n208 = property on="Graphe" class="XYGraph (strict)"("Curseur actif"=u32 0) -> (error out=w199:errorcluster)  [unwired: 2 in, 1 out]
            n209 = property on="Graphe" class="XYGraph (strict)"("Curseur actif"=u32 1) -> (error out=w195:errorcluster)  [unwired: 2 in, 1 out]
            n210 = property on="Graphe" class="XYGraph (strict)"(error in=w199) -> ("Curseur.Indice du curseur"=w197:i32)  [unwired: 1 in, 2 out]
            n211 = property on="Graphe" class="XYGraph (strict)"(error in=w195) -> ("Curseur.Indice du curseur"=w194:i32)  [unwired: 1 in, 2 out]
            n212 = property on="Graphe" class="XYGraph (strict)"() -> ("Cursor.Cursor Plot"=w193:i32)  [unwired: 2 in, 2 out]
            n213 = local read "Graphe"() -> (w192:T1)
            n214 = call "Maths.vi"("Curseur tracé"=w193, "Indice curseur 2"=w194, "Indice curseur 1"=w197, "Graphe"=w192) -> ("Calculs maths"=w189:dbl[])  [unwired: 7 in]
            "Calculs maths" <- w189
            n215 = local read "Selec Maths"() -> (w190:u16)
            n216 = Index Array(array=w189, index=w190) -> (element=w191:dbl)
            n217 = local write "Valeur maths"(w191) -> ()
          }
        }
      }
      event Key Down? {
        n218 = event-data() -> ("PlatMods"=w203:T3)  [unwired: 1 in, 9 out]
        n219 = Unbundle(w203) -> ("Ctrl"=w202:bool)  [unwired: 4 out]
        n220 = property on="Active maths" class="Bool (strict)"() -> ("Valeur"=w201:bool)  [unwired: 2 in, 2 out]
        n221 = And(x=w202, y=w201) -> (x .and. y?=w200:bool)
        n222 = case shown="True" w200 {
          frame False {
          }
          frame True {
            n223 = local read "Calculs maths"() -> (w204:dbl[])
            n224 = call "Affichage calculs maths.vi"("Calculs maths"=w204) -> ()  [unwired: 11 in]
          }
        }
        n225 = event-data() -> ()  [unwired: 2 in, 1 out]
      }
      event "Graphe": Plot Attribute Change {
        n226 = event-data() -> ()  [unwired: 1 in, 8 out]
        n227 = local read "Nbre courbes"() -> (w213:i32)
        n228 = property on="Graphe" class="XYGraph (strict)"() -> ("ActPaletteTool"=w214:i32)  [unwired: 2 in, 2 out]
        n229 = property on="Curseur" class="Ring (strict)"("Strings []"=string[] [] ("Chaînes []")) -> ()  [unwired: 2 in, 2 out]
        n230 = local read "Echelle Y"() -> (w206:u16)
        n231 = Greater?(x=w214, y=u8 1) -> (0:w209:bool)
        n232 = for {
          N: w213 -> [_]
          shift-right: [w243] -> w212
          shift-left: TRUE -> [w242]
          i -> [w240]
          n233 = local read "Tableau de chaînes"() -> (w241:string[])
          n234 = property on="Graphe" class="XYGraph (strict)"("Active Plot"=w240) -> (error out=w244:errorcluster)  [unwired: 2 in, 1 out]
          n235 = property on="Graphe" class="XYGraph (strict)"(error in=w244) -> ("Plot.Visible?"=w238:bool)  [unwired: 1 in, 2 out]
          n236 = Index Array(array=w241, index=w240) -> (element=w239:string)
          n237 = case shown="True" w238 {
            tunnel: w239 -> [_ w247]
            frame False {
            }
            frame True {
              n238 = property on="Curseur" class="Ring (strict)"() -> ("Strings []"=w245:string[])  [unwired: 2 in, 2 out]
              n239 = Array Size(array=w245) -> (size(s)=w246:i32)
              n240 = Insert Into Array(array=w245, index=w246, new element=w247) -> (w248:string[])
              n241 = property on="Curseur" class="Ring (strict)"("Strings []"=w248) -> ()  [unwired: 2 in, 2 out]
            }
          }
          n242 = And(x=w238, y=w242) -> (x .and. y?=w243:bool)
        }
        n243 = Select(t=i8 0 ("cas vrai"), s=w209, f=w206) -> (s? t:f=w210:u16)
        n244 = Select(t=i8 0 ("cas vrai"), s=w209, f=i8 2 ("cas faux")) -> (s? t:f=w216:i8)
        n245 = property on="Graphe" class="XYGraph (strict)"("YScale.ScaleFit"=w210) -> ()  [unwired: 2 in, 2 out]
        n246 = property on="Graphe" class="XYGraph (strict)"("XScale.ScaleFit"=w216) -> ()  [unwired: 2 in, 2 out]
        n247 = flat-sequence {
          tunnel: w212 -> [w218]
          frame #0 {
            n248 = local write "Tout sélectionner"(w218) -> ()
          }
          frame #1 {
            n249 = property on="Curseur" class="Ring (strict)"() -> ("Strings []"=w221:string[])  [unwired: 2 in, 2 out]
            n250 = Index Array(array=w221) -> (element=w222:string)  [unwired: 1 in]
            n251 = Empty String/Path?(string/path=w222) -> (empty?=w220:bool)
            n252 = case shown="False" w220 {
              tunnel: w221 -> [w223 w227]
              tunnel: [w223 w224] -> w219
              frame False {
              }
              frame True {
                n253 = Delete From Array(array=w227, length=1 ("longueur"), index=0 ("indice")) -> (array with subset deleted=w224:string[])  [unwired: 1 out]
              }
            }
            n254 = property on="Curseur" class="Ring (strict)"("Strings []"=w219) -> ()  [unwired: 2 in, 2 out]
          }
          frame #2 {
            n255 = local read "Curseur"() -> (w230:u16)
            n256 = local read "Tableau de chaînes"() -> (w233:string[])
            n257 = property on="Curseur" class="Ring (strict)"() -> ("Strings []"=w231:string[])  [unwired: 2 in, 2 out]
            n258 = Index Array(array=w231, index=w230) -> (element=w232:string)
            n259 = Search 1D Array(1D array=w233, element=w232) -> (index of element=w229:i32)  [unwired: 1 in]
            n260 = property on="Graphe" class="XYGraph (strict)"("Curseur actif"=u32 0) -> (error out=w228:errorcluster)  [unwired: 2 in, 1 out]
            n261 = property on="Graphe" class="XYGraph (strict)"(error in=w228, "Curseur.Tracé du curseur"=w229) -> ()  [unwired: 1 in, 2 out]
          }
          frame #3 {
            n262 = property on="Graphe" class="XYGraph (strict)"() -> ("Cursor.Cursor Y"=w235:dbl)  [unwired: 2 in, 2 out]
            n263 = property on="Graphe" class="XYGraph (strict)"() -> ("Cursor.Cursor X"=w237:dbl)  [unwired: 2 in, 2 out]
            n264 = local write "Y"(w235) -> ()
            n265 = To Time Stamp(1:w237) -> (0:w236:timestamp)
            n266 = local write "X"(w236) -> ()
          }
        }
      }
      event "Tout sélectionner": Value Change {
        n267 = event-data() -> ("NewVal"=w262:bool)  [unwired: 1 in, 5 out]
        n268 = flat-sequence {
          frame #0 {
            n269 = local read "Nbre courbes"() -> (w264:i32)
            n270 = for {
              N: w264 -> [_]
              i -> [w266]
              n271 = property on="Graphe" class="XYGraph (strict)"("Active Plot"=w266) -> (error out=w267:errorcluster)  [unwired: 2 in, 1 out]
              n272 = property on="Graphe" class="XYGraph (strict)"(error in=w267, "Plot.Visible?"="Tout sélectionner") -> ()  [unwired: 1 in, 2 out]
            }
          }
          frame #1 {
            n273 = property on="Graphe" class="XYGraph (strict)"() -> ("ActPaletteTool"=w268:i32)  [unwired: 2 in, 2 out]
            n274 = local read "Echelle Y"() -> (w274:u16)
            n275 = property on="Graphe" class="XYGraph (strict)"("YScale.ScaleFit"=w274) -> ()  [unwired: 2 in, 2 out]
            n276 = Greater?(x=w268, y=u8 1) -> (0:w270:bool)
            n277 = Select(t=i8 0 ("cas vrai"), s=w270, f=i8 2 ("cas faux")) -> (s? t:f=w271:i8)
            n278 = property on="Graphe" class="XYGraph (strict)"("XScale.ScaleFit"=w271) -> ()  [unwired: 2 in, 2 out]
          }
        }
        n279 = case shown="True" w262 {
          tunnel: [_ w263] -> w249
          frame False {
          }
          frame True {
            n280 = local read "Tableau de chaînes"() -> (w263:string[])
          }
        }
        n281 = local read "Curseur"() -> (w252:u16)
        n282 = property on="Curseur" class="Ring (strict)"("Strings []"=w249) -> ()  [unwired: 2 in, 2 out]
        n283 = Index Array(array=w249, index=w252) -> (element=w251:string)
        n284 = Search 1D Array(1D array=w249, element=w251) -> (index of element=w258:i32)  [unwired: 1 in]
        n285 = property on="Graphe" class="XYGraph (strict)"("Curseur actif"=u32 0) -> (error out=w260:errorcluster)  [unwired: 2 in, 1 out]
        n286 = property on="Graphe" class="XYGraph (strict)"(error in=w260, "Cursor.CursorMode"=u32 1 ("Curseur.Mode du curseur")) -> (error out=w261:errorcluster)  [unwired: 1 in, 1 out]
        n287 = property on="Graphe" class="XYGraph (strict)"(error in=w261, "Curseur.Tracé du curseur"=w258) -> (error out=w253:errorcluster)  [unwired: 1 in, 1 out]
        n288 = property on="Graphe" class="XYGraph (strict)"(error in=w253) -> (error out=w254:errorcluster, "Cursor.Cursor X"=w257:dbl)  [unwired: 1 in, 1 out]
        n289 = To Time Stamp(1:w257) -> (0:w256:timestamp)
        n290 = local write "X"(w256) -> ()
        n291 = property on="Graphe" class="XYGraph (strict)"(error in=w254) -> ("Cursor.Cursor Y"=w255:dbl)  [unwired: 1 in, 2 out]
        n292 = local write "Y"(w255) -> ()
      }
      event "Quitter graphe": Value Change {
        n293 = event-data() -> ("NewVal"=w275:bool)  [unwired: 1 in, 5 out]
        n294 = invoke on="Tableau de chaînes" class="Tabl (strict)" method="Reinit To Default"() -> ()  [unwired: 3 in, 3 out]
      }
      event "Bouton Aide": Value Change {
        n295 = event-data() -> ()  [unwired: 1 in, 6 out]
        n296 = call <vilib>:"Application Directory.vi"() -> ("Application Directory"=w277:path)
        n297 = Build Path(base path=w277, name or relative path="Logiciel GRAPHE_Instruction.pdf" ("standard input")) -> (appended path=w276:path)
        n298 = call "Open PDF.vi"("Path"=w276) -> ()  [unwired: 5 in, 2 out]
      }
    }
  }
  n299 = local write "Echelle Y"(w22) -> ()
  n300 = property on="Mini" class="DigNum (strict)"("DisabledEnum"=w22) -> ()  [unwired: 2 in, 2 out]
  n301 = property on="Maxi" class="DigNum (strict)"("DisabledEnum"=w22) -> ()  [unwired: 2 in, 2 out]
  n302 = local write "X"(timestamp(0 s since 1904-01-01) ("X")) -> ()
  n303 = for {
    tunnel: "Tableau de chaînes" -> [w282] mode=indexing
    tunnel: [w279] -> w4
    i -> [w285]
    n304 = property on="Graphe" class="XYGraph (strict)"("LegAutosize"=TRUE ("Légende:Redimensionnement automatique")) -> (error out=w280:errorcluster)  [unwired: 2 in, 1 out]
    n305 = property on="Graphe" class="XYGraph (strict)"(error in=w280, "Active Plot"=w285) -> (error out=w286:errorcluster)  [unwired: 1 in, 1 out]
    n306 = property on="Graphe" class="XYGraph (strict)"(error in=w286, "Plot.Visible?"=TRUE ("Tracé.Visible")) -> (error out=w283:errorcluster)  [unwired: 1 in, 1 out]
    n307 = property on="Graphe" class="XYGraph (strict)"(error in=w283, "Plot.Plot Name"=w282) -> (error out=w279:errorcluster)  [unwired: 1 in, 1 out]
  }
  n308 = property on="Active maths" class="Bool (strict)"("Valeur"=FALSE ("Valeur (Signalisation)")) -> ()  [unwired: 2 in, 2 out]
  n309 = property on="Graphe" class="XYGraph (strict)"(error in=w4, "LegAutosize"=FALSE ("Légende:Redimensionnement automatique")) -> (error out=w6:errorcluster)  [unwired: 1 in, 1 out]
  n310 = property on="Graphe" class="XYGraph (strict)"(error in=w6, "LegPos"=T2 {"Left"=804, "Top"=34} ("Légende:Position")) -> (error out=w5:errorcluster)  [unwired: 1 in, 1 out]
  n311 = Array Size(array="Tableau de chaînes") -> (size(s)=w12:i32)
  "Nbre courbes" <- w12
  n312 = Greater?(x=w12, y=w13) -> (0:w14:bool)
  n313 = property on="Graphe" class="XYGraph (strict)"(error in=w5, "LegPlotMin"=w12) -> (error out=w15:errorcluster)  [unwired: 1 in, 1 out]
  n314 = Select(t=w13, s=w14, f=w12) -> (s? t:f=w11:i32)
  n315 = property on="Graphe" class="XYGraph (strict)"(error in=w15, "LegNumRows"=w11) -> (error out=w1:errorcluster)  [unwired: 1 in, 1 out]
  n316 = flat-sequence {
    tunnel: [w288] -> w2
    tunnel: w1 -> [w288]
    frame #0 {
      n317 = Wait (ms)(milliseconds to wait=u32 500 ("attente (ms)")) -> ()  [unwired: 1 out]
    }
  }
  n318 = property on="Graphe" class="XYGraph (strict)"(error in=w2, "LegAutosize"=TRUE ("Légende:Redimensionnement automatique")) -> ()  [unwired: 1 in, 2 out]
  "Valeur maths" <- 0.0 ("Valeur maths")
